vi "getInheritanceChain.vi"(8 "error in (no error)":errorcluster, 11 "LinkedList in":refnum<class "LinkedList.lvclass">) -> (0 "error out":errorcluster, 2 "Inheritance Chain":string[](array[string]), 3 "LinkedList out":refnum<class "LinkedList.lvclass">)   [LabVIEW 2009, in "LinkedList.lvclass"]
doc: "Returns the inheritance chain."
uses:
  LinkedList.lvclass
  Structure/Structure.lvclass
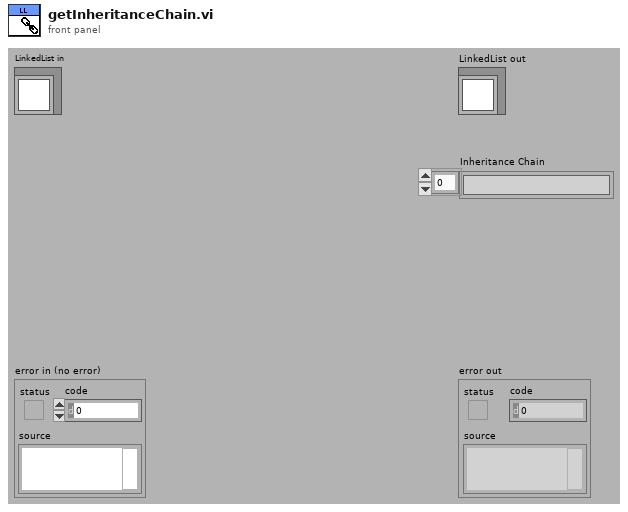
[diagram p1: front panel]
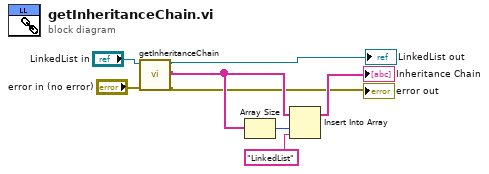
[diagram p0: block diagram]
diagram:
  n1 = call-parent "getInheritanceChain.vi"("error in (no error)"="error in (no error)", "Structure in"="LinkedList in") -> ("error out"=→"error out":errorcluster, "Inheritance Chain"=w4:string[], "Structure out"=→"LinkedList out":refnum<class "LinkedList.lvclass">)  [unwired: 7 in]
  n2 = Array Size(array=w4) -> (size(s)=w6:i32)
  n3 = Insert Into Array(array=w4, index=w6, new element="LinkedList") -> (→"Inheritance Chain":string[])
